vi "Calc Destination Yaw.vi"(9 "Angle to add":dbl, 10 "Current yaw":dbl) -> (2 "Destiantion yaw":dbl)   [LabVIEW 2014]
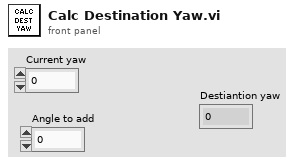
[diagram p1: front panel]
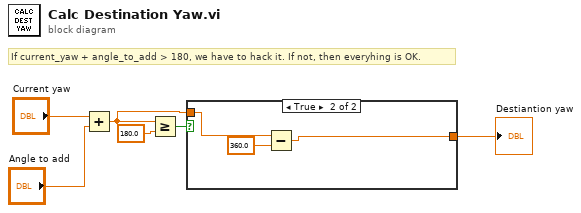
[diagram p0: block diagram]
diagram:
  # "If current_yaw + angle_to_add > 180, we have to hack it. If not, then everyhing is OK."
  n1 = Add(x="Current yaw", y="Angle to add") -> (x+y=w2:dbl)
  n2 = Greater Or Equal?(x=w2, y=180.0) -> (x >= y?=w3:bool)
  n3 = case shown="True" w3 {
    tunnel: w2 -> [w7 w10]
    tunnel: [w7 w8] -> w1
    frame False {
    }
    frame True {
      n4 = Subtract(x=w10, y=360.0) -> (x-y=w8:dbl)
    }
  }
  "Destiantion yaw" <- w1
